vi "Write Previous Pattern Path.vi"(8 "error in (no error)":errorcluster, 10 "Previous Pattern Path":path, 11 "DMD in":refnum<class "DMD.lvclass">) -> (0 "error out":errorcluster, 3 "DMD out":refnum<class "DMD.lvclass">)   [LabVIEW 2013, in "DMD.lvclass"]
uses:
  DMD.lvclass
  DMD.lvclass/DMD.ctl
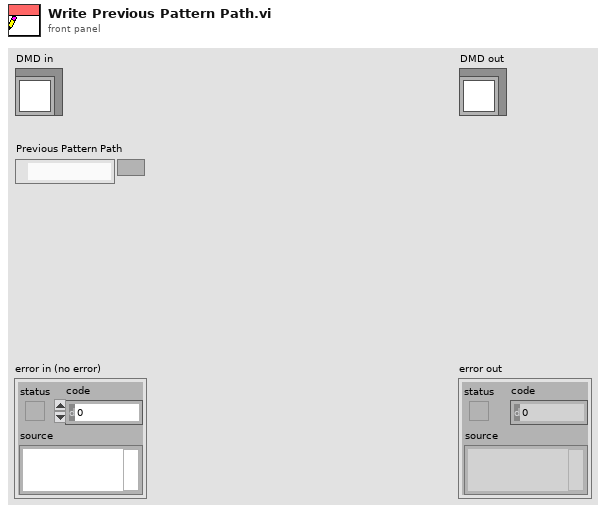
[diagram p1: front panel]
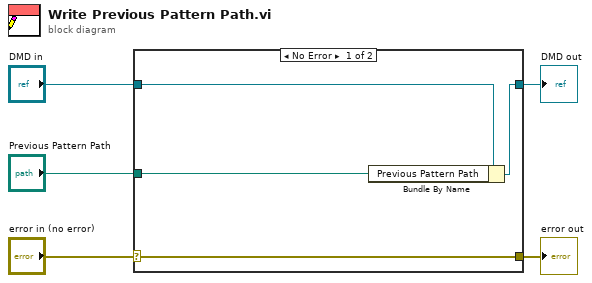
[diagram p0: block diagram]
diagram:
  n1 = case shown="No Error" "error in (no error)" {
    selector: "error in (no error)" -> [w9 w10]
    tunnel: [w9 w10] -> w4
    tunnel: [w7 w11] -> w2
    tunnel: "DMD in" -> [w8 w11]
    tunnel: "Previous Pattern Path" -> [w6 _]
    frame No Error {
      n2 = Bundle By Name(cluster=w8, "Previous Pattern Path"=w6) -> (w7:refnum<class "DMD.lvclass">)
    }
    frame Error {
    }
  }
  "error out" <- w4
  "DMD out" <- w2
